vi "Odometry_omni.vi"(6 "Reset":bool, 8 "parameter":T1={"wheel radius(cm)"=4.8, "encoder conunts/rev"=6144.0, "wheel distance(cm)"=14.0}, 11 "Encoder-in":dbl[](array[numeric])) -> (2 "now [X,Y,theta] (cm,cm,deg)":cluster{"X":dbl, "Y":dbl, "theta (deg)":dbl})   [LabVIEW 2019]
doc: "Odometry of 2-wheel (output-cm)\nsystem sonstants:\nradius of wheel 0.197 m , encoder counts 2000 , gear ratio 26 , pulley ratio 26/36\ntwo wheel distance 0.45m\n\nencoder in 0-encoder1(right) 1-encoder2(left)\n\nwrited by Wei-Shun Yu"
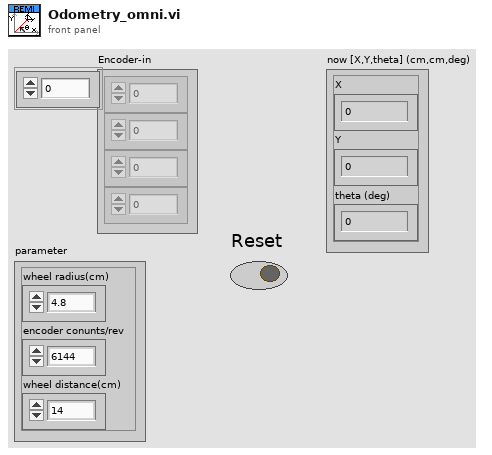
[diagram p1: front panel]
types:
  T1 = cluster{"wheel radius(cm)":dbl, "encoder conunts/rev":dbl, "wheel distance(cm)":dbl}
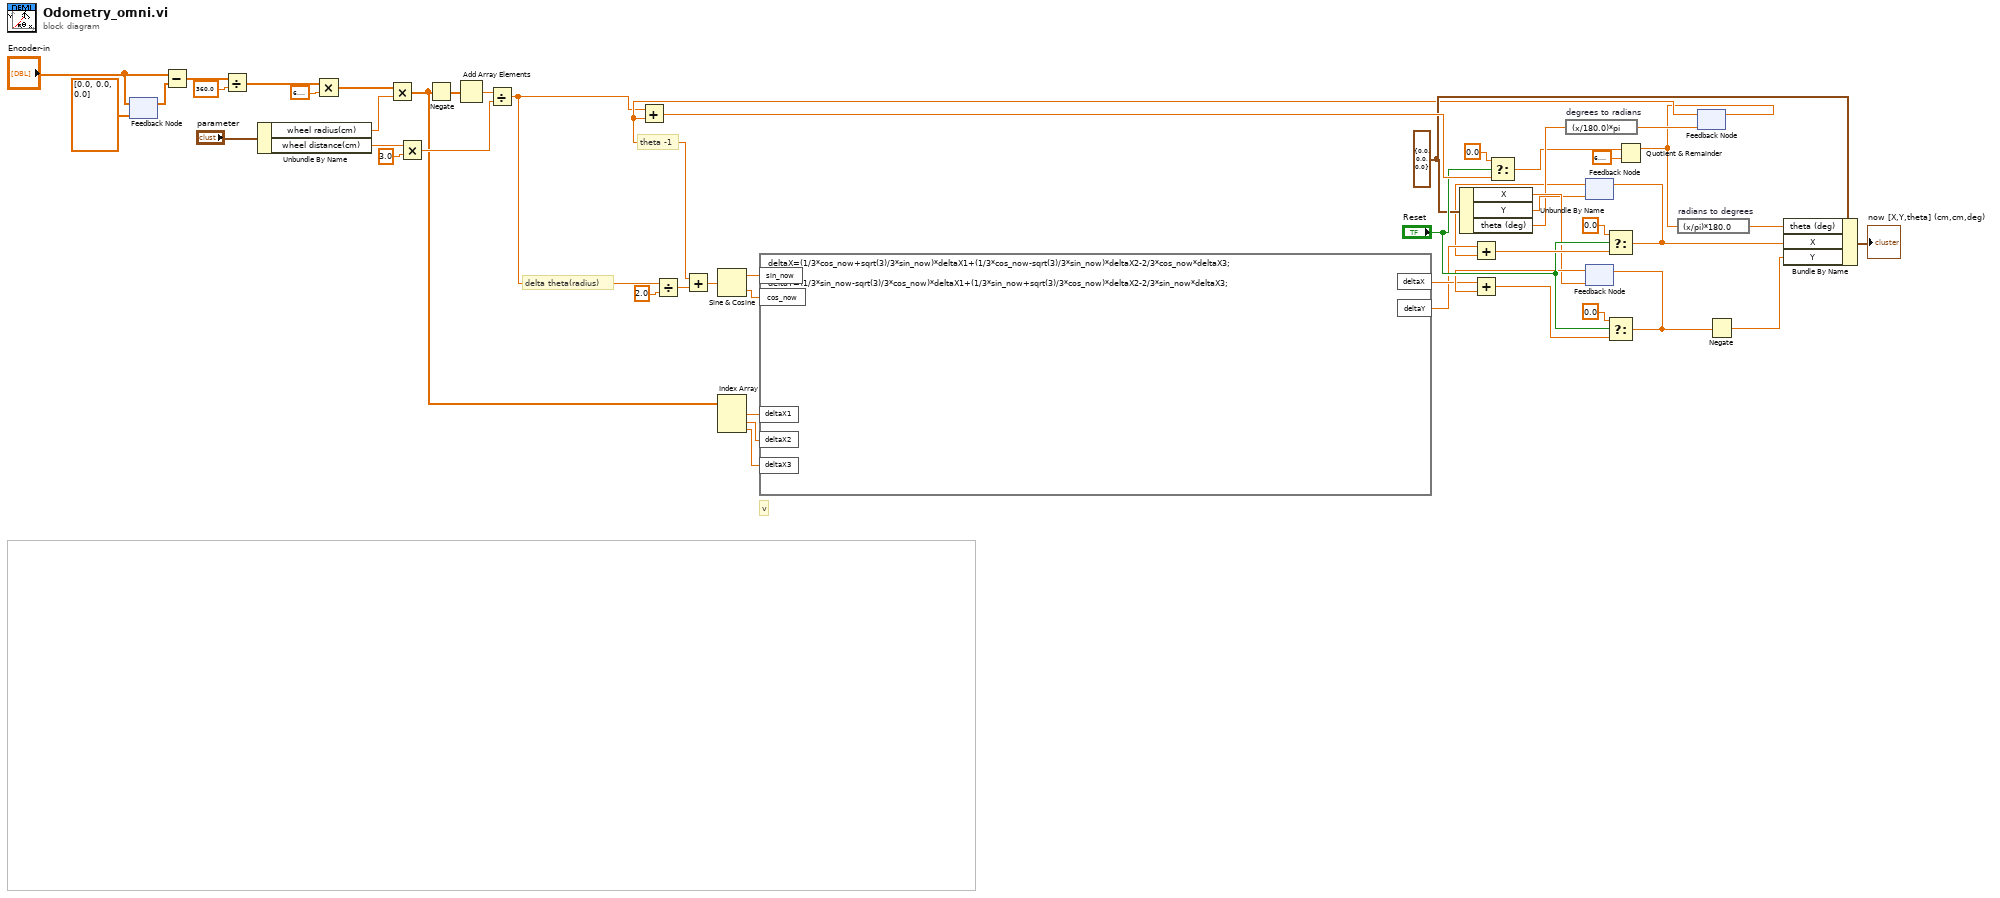
[diagram p0: block diagram]
diagram:
  w10 = cluster{"X":dbl, "Y":dbl, "theta (deg)":dbl} {"X"=0.0, "Y"=0.0, "theta (deg)"=0.0} ("init x y theta")
  # "v"
  # "theta -1"
  # "delta theta(radius)"
  n1 = feedback-in #1("Encoder-in") -> ()
  n2 = feedback #1(dbl[] [0.0, 0.0, 0.0] ("Encoder-in")) -> (w38:dbl[])
  n3 = Subtract(x="Encoder-in", y=w38) -> (x-y=w36:dbl[])
  n4 = Divide(x=w36, y=360.0) -> (x/y=w35:dbl[])
  n5 = Unbundle By Name("parameter") -> ("wheel radius(cm)"=w32:dbl, "wheel distance(cm)"=w29:dbl)
  n6 = Multiply(x=w35, y=6.283185307179586) -> (x*y=w33:dbl[])
  n7 = Multiply(x=w33, y=w32) -> (x*y=w25:dbl[])
  n8 = Multiply(x=w29, y=3.0) -> (x*y=w27:dbl)
  n9 = Negate(x=w25) -> (-x=w31:dbl[])
  n10 = Add Array Elements(numeric array=w31) -> (sum=w30:dbl)
  n11 = Divide(x=w30, y=w27) -> (x/y=w7:dbl)
  n12 = Divide(x=w7, y=2.0) -> (x/y=w23:dbl)
  n13 = Index Array(array=w25) -> (element #1=w22:dbl, element #2=w21:dbl, element #3=w20:dbl)  [unwired: 3 in]
  n14 = Unbundle By Name(w10) -> ("X"=w15:dbl, "Y"=w14:dbl, "theta (deg)"=w6:dbl)
  n15 = expression code="(x/180.0)*pi" "degrees to radians"(w6) -> (w5:dbl)
  n16 = feedback #2(w14) -> (w1:dbl)
  n17 = feedback #3(w15) -> (w46:dbl)
  n18 = feedback #4(w5) -> (w8:dbl)
  n19 = Add(x=w7, y=w8) -> (x+y=w48:dbl)
  n20 = Add(x=w8, y=w23) -> (x+y=w26:dbl)
  n21 = Sine & Cosine(0:w26) -> (1:w41:dbl, 2:w40:dbl)
  n22 = formula code="deltaX=(1/3*cos_now+sqrt(3)/3*sin_now)*deltaX1+(1/3*cos_now-sqrt(3)/3*sin_now)*deltaX2-2/3*cos_now*deltaX3;\n\ndeltaY=(1/3*sin_now-sqrt(3)/3*cos_now)*deltaX1+(1/3*sin_now+sqrt(3)/3*cos_now)*deltaX2-2/3*sin_now*deltaX3;"("sin_now"=w41, "cos_now"=w40, "deltaX1"=w22, "deltaX2"=w21, "deltaX3"=w20) -> ("deltaX"=w19:dbl, "deltaY"=w18:dbl)
  n23 = Add(x=w18, y=w1) -> (x+y=w49:dbl)
  n24 = Add(x=w19, y=w46) -> (x+y=w50:dbl)
  n25 = Select(t=0.0, s="Reset", f=w48) -> (s? t:f=w4:dbl)
  n26 = Select(t=0.0, s="Reset", f=w49) -> (s? t:f=w13:dbl)
  n27 = feedback-in #2(w13) -> ()
  n28 = Select(t=0.0, s="Reset", f=w50) -> (s? t:f=w12:dbl)
  n29 = feedback-in #3(w12) -> ()
  n30 = Quotient & Remainder(x=w4, y=6.283185307179586) -> (x-y*floor(x/y)=w2:dbl)  [unwired: 1 out]
  n31 = expression code="(x/pi)*180.0" "radians to degrees"(w2) -> (w17:dbl)
  n32 = feedback-in #4(w2) -> ()
  n33 = Negate(x=w12) -> (-x=w11:dbl)
  n34 = Bundle By Name(cluster=w10, "theta (deg)"=w17, "X"=w13, "Y"=w11) -> (→"now [X,Y,theta] (cm,cm,deg)":cluster{"X":dbl, "Y":dbl, "theta (deg)":dbl})
